vi "EN String Values.vi"(10 "Label.Text":string, 11 "UserInputs":T1) -> (3 "String":string)   [LabVIEW 2011]
uses:
  user project design.ctl
panel:
  out "label":string[](array[string])
  out "String":string[](array[string])
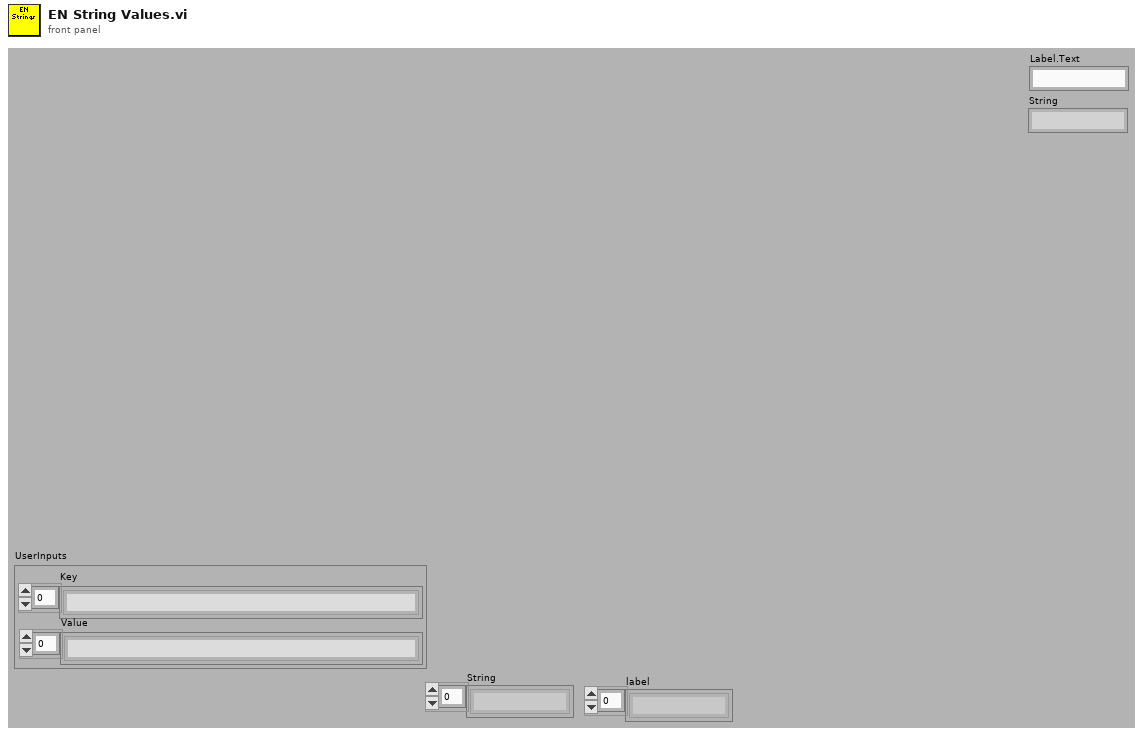
[diagram p1: front panel]
types:
  T1 = typedef "user project design.ctl" = cluster{"Key":string[], "Value":string[]}
  T2 = typedef "AguaClara Library.lvlib/User Information.ctl" = cluster{"First Name":string, "Last Name":string, "Email Address":string, "Organization":string, "Language":enum16{"English", "Español", "French"}, "Country":T3}
  T3 = typedef "Country Ring.ctl" = u16
  T4 = typedef "AguaClara Library.lvlib/Basic Inputs.ctl" = cluster{"Q.Plant":dbl[unit], "C.CoagDoseMax":dbl[unit], "C.CoagStock":dbl[unit], "Ti.CoagStock":dbl[unit], "EN.DrillSeries":enum16{"English", "Metric"}, "EN.TubeSeries":enum16{"English", "Metric"}, "N.SedTanks":dbl, "N.SedBaysEst":dbl, "W.SedPlate":dbl[unit], "L.SedPlateSheet":dbl[unit], "T.SedPlate":dbl[unit], "T.PlantWall":dbl[unit], "H.FlocOption":dbl[unit], "T.FlocBaffleRigidH":dbl[unit], "T.ConcreteMin":dbl[unit], "T.SedWeir":dbl[unit], "T.FlocBaffleRigidV":dbl[unit]}
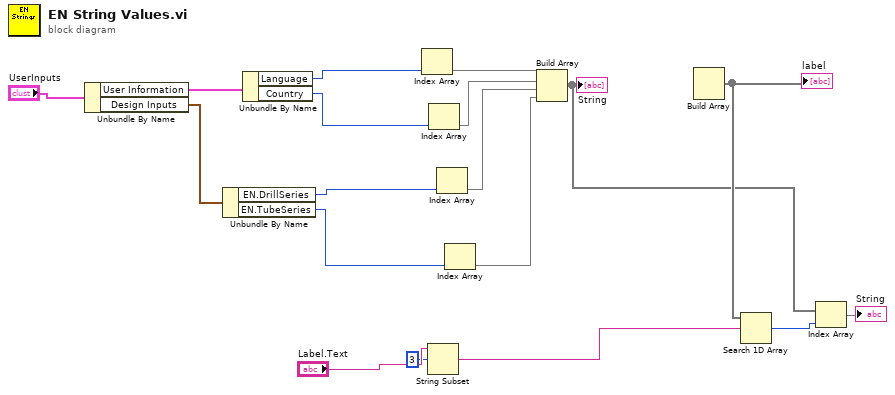
[diagram p0: block diagram]
diagram:
  n1 = Unbundle By Name("UserInputs") -> ("User Information"=w21:T2, "Design Inputs"=w20:T4)
  n2 = Unbundle By Name(w20) -> ("EN.DrillSeries"=w17:enum16{"English", "Metric"}, "EN.TubeSeries"=w16:enum16{"English", "Metric"})
  n3 = Unbundle By Name(w21) -> ("Language"=w19:enum16{"English", "Español", "French"}, "Country"=w18:T3)
  n4 = Index Array(index=w19) -> (element=w15)  [unwired: 1 in]
  n5 = String Subset(string="Label.Text", offset (0)=3) -> (substring=w5:string)  [unwired: 1 in]
  n6 = Index Array(index=w18) -> (element=w14)  [unwired: 1 in]
  n7 = Index Array(index=w17) -> (element=w13)  [unwired: 1 in]
  n8 = Index Array(index=w16) -> (element=w12)  [unwired: 1 in]
  n9 = Build Array(w15, w14, w13, w12) -> (w3:void[])
  "String" <- w3
  n10 = Build Array() -> (w4:void[], w11:dbl, w10:dbl, w9:dbl, w8:dbl)
  "label" <- w4
  n11 = Search 1D Array(1D array=w4, element=w5) -> (index of element=w2:i32)  [unwired: 1 in]
  n12 = Index Array(array=w3, index=w2) -> (element=→"String")
